vi "Disconnect.vi"(8 "error in":errorcluster, 11 "6700C in":refnum<class "6700C.lvclass">) -> (0 "error out":errorcluster, 3 "6700C out":refnum<class "6700C.lvclass">)   [LabVIEW 2019, in "6700C.lvlib" / "6700C.lvclass"]
uses:
  Library/6700C.lvclass
  Library/6700C.lvclass/6700C.ctl
  <instrlib>/Agilent N6700 Series/Agilent N6700 Series.lvlib
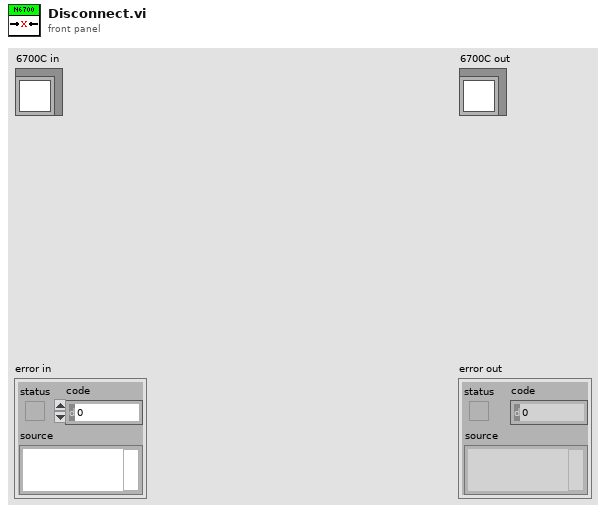
[diagram p1: front panel]
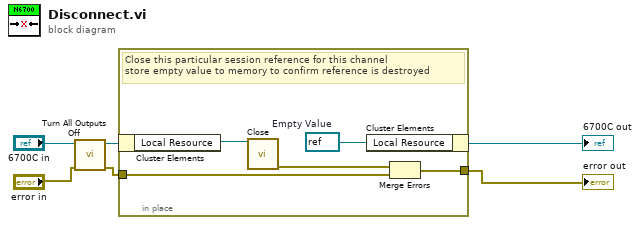
[diagram p0: block diagram]
diagram:
  n1 = call "Turn All Outputs Off.vi"("error in"="error in", "6700C in"="6700C in") -> ("error out"=w1:errorcluster, "6700C out"=w2:refnum<class "6700C.lvclass">)  [unwired: 8 in]
  n2 = in-place {
    in-place-border: w1 -> [w8]
    in-place-border: [w7] -> w3
    w10 = refnum<visa-resource-name> refnum  # Empty Value
    # "Close this particular session reference for this channel\nstore empty value to memory to confirm reference is destroyed"
    n3 = in-place-cluster #1(w2) -> ("Local Resource"=w11:refnum<visa-resource-name>)
    n4 = call <instrlib>:"Close.vi"("VISA resource name"=w11) -> ("error out"=w9:errorcluster)  [unwired: 14 in]
    n5 = in-place-cluster #1("Local Resource"=w10) -> (→"6700C out":refnum<class "6700C.lvclass">)
    n6 = Merge Errors(w9, w8) -> (w7:errorcluster)
  }
  "error out" <- w3
